vi "OGB Replace Keyword in String.vi"(1 "Value":string, 2 "Keyword":string, 3 "String":string) -> (0 "String out":string)   [LabVIEW 2011]
panel:
  out "error out":errorcluster
  in  "error in (no error)":errorcluster
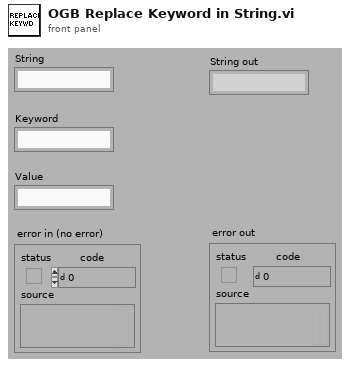
[diagram p1: front panel]
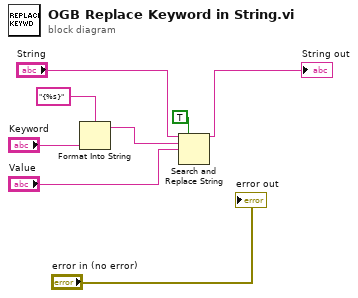
[diagram p0: block diagram]
diagram:
  n1 = Format Into String(format string="{%s}", "Keyword") -> (resulting string=w6:string)  [unwired: 2 in, 1 out]
  n2 = Search and Replace String(replace all?=TRUE ("replace all? (F)"), input string="String", search string=w6, replace string="Value") -> (result string=→"String out":string)  [unwired: 4 in, 3 out]
  "error out" <- "error in (no error)"
